vi "SetPersistentConfiguration.vi"(8 "Error In":errorcluster, 9 "DataIn":variant, 11 "reference in":refnum<class "TAFBaseGUI.lvclass">) -> (0 "Error Out":errorcluster, 1 "DataOut":variant, 3 "reference out":refnum<class "TAFBaseGUI.lvclass">)   [LabVIEW 2021, in "TAFBaseGUI.lvclass"]
uses:
  TAFBaseGUI.lvclass
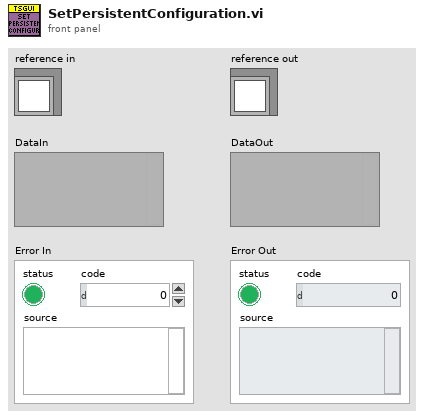
[diagram p1: front panel]
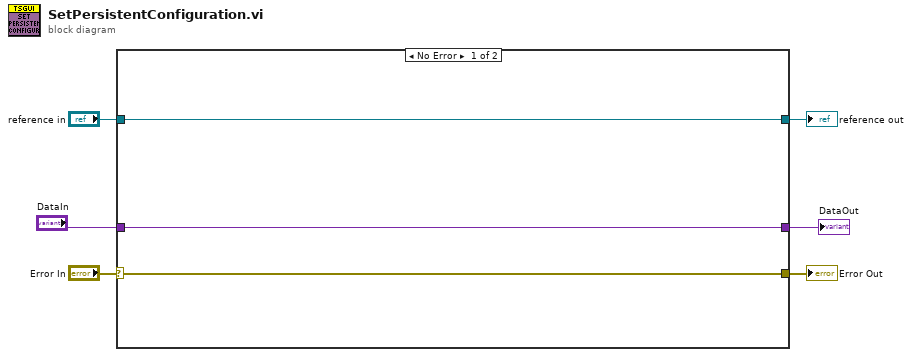
[diagram p0: block diagram]
diagram:
  n1 = case shown="No Error" "Error In" {
    selector: "Error In" -> [w7 w12]
    tunnel: [w7 w12] -> w5
    tunnel: [w9 w11] -> w3
    tunnel: "reference in" -> [w9 w11]
    tunnel: [w8 w10] -> w2
    tunnel: "DataIn" -> [w8 w10]
    frame No Error {
    }
    frame Error {
    }
  }
  "Error Out" <- w5
  "reference out" <- w3
  "DataOut" <- w2
